vi "test_case_selection_of_indexes_of_nonzero_elements.vi"() -> ()   [LabVIEW 2020]
uses:
  <vilib>/Waveform/DWDTOps.llb/Digital Pattern Generator (Random).vi
  <vilib>/Waveform/DWDTOps.llb/DWDT Digital to Boolean Array.vi
panel:
  out "CHANNEL_0":i32[][](array[numeric])
  out "CHANNEL_1":i32[][](array[numeric])
  out "CHANNEL_2":i32[][](array[numeric])
  out "CHANNEL_3":i32[][](array[numeric])
  out "CHANNEL_4":i32[][](array[numeric])
  out "CHANNEL_5":i32[][](array[numeric])
  out "CHANNEL_6":i32[][](array[numeric])
  out "CHANNEL_7":i32[][](array[numeric])
  out "INPUT_STREAM":bool[][](array[boolean]) caption="tableau de booléens"
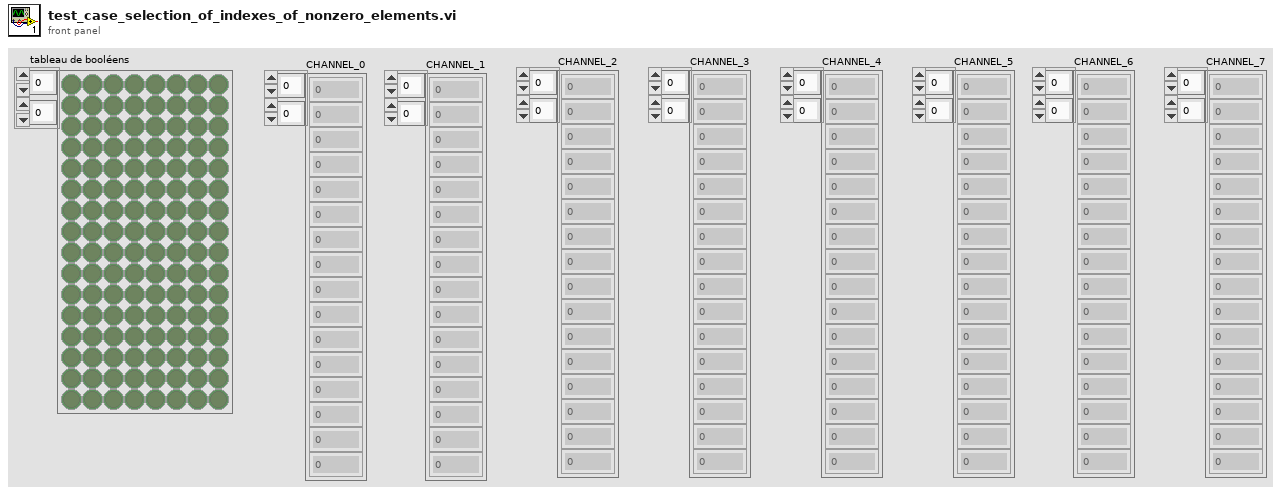
[diagram p1: front panel]
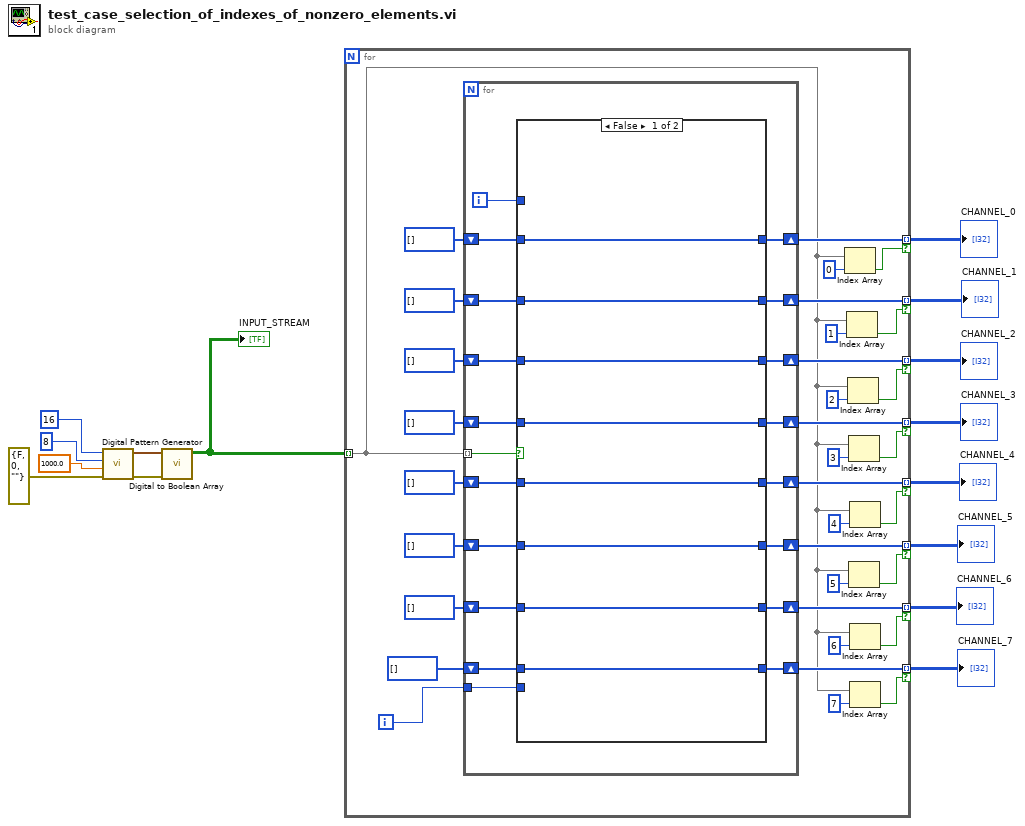
[diagram p0: block diagram]
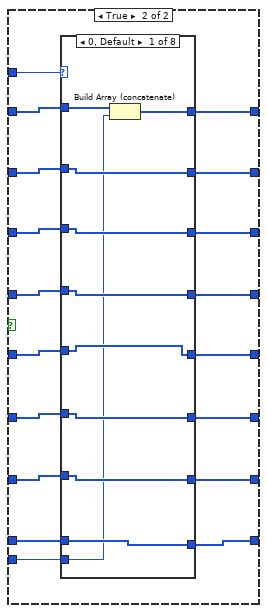
[diagram p2: hidden frame]
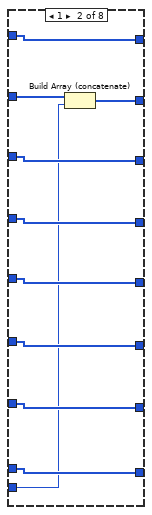
[diagram p3: hidden frame]
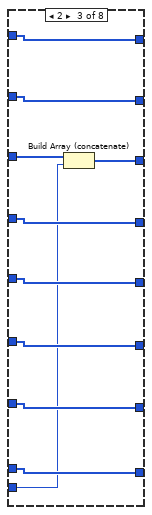
[diagram p4: hidden frame]
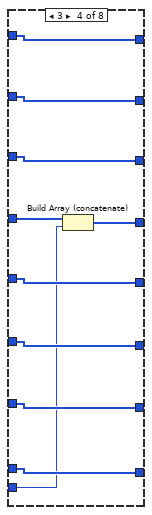
[diagram p5: hidden frame]
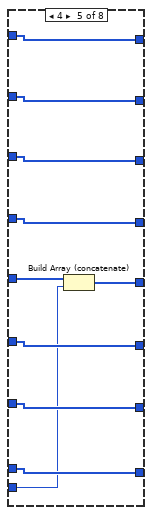
[diagram p6: hidden frame]
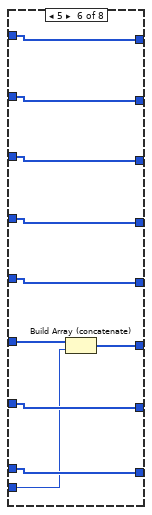
[diagram p7: hidden frame]
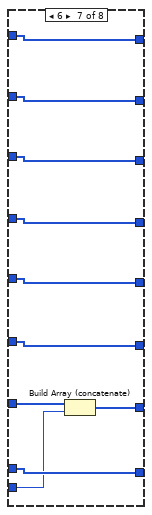
[diagram p8: hidden frame]
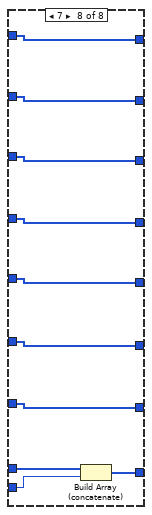
[diagram p9: hidden frame]
diagram:
  n1 = call-poly <vilib>:"Digital Pattern Generator.vi"("error in (no error)"=errorcluster {"status"=FALSE, "code"=0, "source"=""}, "sample rate"=1000.0, "number of signals"=u32 8, "number of samples"=u32 16) -> ("error out"=w10:errorcluster, "digital waveform"=w12:digitalwaveform)  [unwired: 6 in]
  n2 = call-poly <vilib>:"Digital to Boolean Array.vi"("error in (no error)"=w10, "digital waveform"=w12) -> ("boolean array"=w9:bool[][])  [unwired: 8 in, 1 out]
  "INPUT_STREAM" <- w9
  n3 = for {
    tunnel: w9 -> [w29] mode=indexing
    tunnel: [w48] -> w8 mode=indexing if=w23
    tunnel: [w46] -> w7 mode=indexing if=w24
    tunnel: [w45] -> w6 mode=indexing if=w25
    tunnel: [w44] -> w5 mode=indexing if=w26
    tunnel: [w43] -> w4 mode=indexing if=w27
    tunnel: [w42] -> w3 mode=indexing if=w28
    tunnel: [w41] -> w2 mode=indexing if=w30
    tunnel: [w40] -> w1 mode=indexing if=w31
    i -> [w49]
    n4 = for {
      tunnel: w49 -> [w67]
      tunnel: w29 -> [w64] mode=indexing
      shift-right: [w66] -> w48
      shift-left: i32[] [] -> [w65]
      shift-right: [w63] -> w46
      shift-left: i32[] [] -> [w62]
      shift-right: [w61] -> w45
      shift-left: i32[] [] -> [w60]
      shift-right: [w59] -> w44
      shift-left: i32[] [] -> [w58]
      shift-right: [w57] -> w43
      shift-left: i32[] [] -> [w56]
      shift-right: [w55] -> w42
      shift-left: i32[] [] -> [w54]
      shift-right: [w53] -> w41
      shift-left: i32[] [] -> [w52]
      shift-right: [w51] -> w40
      shift-left: i32[] [] -> [w50]
      i -> [w68]
      n5 = case shown="False" w64 {
        tunnel: w68 -> [_ w94]
        tunnel: w67 -> [_ w93]
        tunnel: [w76 w92] -> w66
        tunnel: w65 -> [w76 w91]
        tunnel: [w69 w90] -> w63
        tunnel: w62 -> [w69 w89]
        tunnel: [w70 w88] -> w61
        tunnel: w60 -> [w70 w87]
        tunnel: [w71 w86] -> w59
        tunnel: w58 -> [w71 w85]
        tunnel: [w72 w84] -> w57
        tunnel: w56 -> [w72 w83]
        tunnel: [w73 w82] -> w55
        tunnel: w54 -> [w73 w81]
        tunnel: [w74 w80] -> w53
        tunnel: w52 -> [w74 w79]
        tunnel: [w75 w78] -> w51
        tunnel: w50 -> [w75 w77]
        frame False {
        }
        frame True {
          n6 = case shown="0, Default" w94 {
            tunnel: w93 -> [w97 w108 w119 w130 w141 w152 w163 w174]
            tunnel: [w104 w114 w124 w134 w144 w154 w164 w173] -> w92
            tunnel: w91 -> [w104 w114 w124 w134 w144 w154 w164 w172]
            tunnel: [w103 w113 w123 w133 w143 w153 w162 w171] -> w90
            tunnel: w89 -> [w103 w113 w123 w133 w143 w153 w161 w171]
            tunnel: [w102 w112 w122 w132 w142 w151 w160 w170] -> w88
            tunnel: w87 -> [w102 w112 w122 w132 w142 w150 w160 w170]
            tunnel: [w101 w111 w121 w131 w140 w149 w159 w169] -> w86
            tunnel: w85 -> [w101 w111 w121 w131 w139 w149 w159 w169]
            tunnel: [w100 w110 w120 w129 w138 w148 w158 w168] -> w84
            tunnel: w83 -> [w100 w110 w120 w128 w138 w148 w158 w168]
            tunnel: [w99 w109 w118 w127 w137 w147 w157 w167] -> w82
            tunnel: w81 -> [w99 w109 w117 w127 w137 w147 w157 w167]
            tunnel: [w98 w107 w116 w126 w136 w146 w156 w166] -> w80
            tunnel: w79 -> [w98 w106 w116 w126 w136 w146 w156 w166]
            tunnel: [w96 w105 w115 w125 w135 w145 w155 w165] -> w78
            tunnel: w77 -> [w95 w105 w115 w125 w135 w145 w155 w165]
            frame 0, Default {
              n7 = Build Array (concatenate)(w95, w97) -> (w96:i32[])
            }
            frame 1 {
              n8 = Build Array (concatenate)(w106, w108) -> (w107:i32[])
            }
            frame 2 {
              n9 = Build Array (concatenate)(w117, w119) -> (w118:i32[])
            }
            frame 3 {
              n10 = Build Array (concatenate)(w128, w130) -> (w129:i32[])
            }
            frame 4 {
              n11 = Build Array (concatenate)(w139, w141) -> (w140:i32[])
            }
            frame 5 {
              n12 = Build Array (concatenate)(w150, w152) -> (w151:i32[])
            }
            frame 6 {
              n13 = Build Array (concatenate)(w161, w163) -> (w162:i32[])
            }
            frame 7 {
              n14 = Build Array (concatenate)(w172, w174) -> (w173:i32[])
            }
          }
        }
      }
    }
    n15 = Index Array(array=w29, index=0 ("indice")) -> (element=w31:bool)
    n16 = Index Array(array=w29, index=1 ("indice")) -> (element=w30:bool)
    n17 = Index Array(array=w29, index=2 ("indice")) -> (element=w28:bool)
    n18 = Index Array(array=w29, index=3 ("indice")) -> (element=w27:bool)
    n19 = Index Array(array=w29, index=5 ("indice")) -> (element=w25:bool)
    n20 = Index Array(array=w29, index=4 ("indice")) -> (element=w26:bool)
    n21 = Index Array(array=w29, index=6 ("indice")) -> (element=w24:bool)
    n22 = Index Array(array=w29, index=7 ("indice")) -> (element=w23:bool)
  }
  "CHANNEL_7" <- w8
  "CHANNEL_6" <- w7
  "CHANNEL_5" <- w6
  "CHANNEL_4" <- w5
  "CHANNEL_3" <- w4
  "CHANNEL_2" <- w3
  "CHANNEL_1" <- w2
  "CHANNEL_0" <- w1
